vi "f_6_Eon.vi"(0 "file path (IN)":path, 1 "Project #":string, 2 "Request #":string, 3 "TEST #":string, 5 "error in (no error)":errorcluster, 6 "VGE":dbl, 8 "VCE":dbl) -> (14 "file path (OUT)":path, 15 "Eon (uj)":dbl, 16 "DONE Eon":bool, 19 "error out":errorcluster)   [LabVIEW 2020]
uses:
  GlobIndSw1.vi
  <vilib>/Waveform/WDTOps.llb/WDT Waveform Duration DBL.vi
  <vilib>/Waveform/WDTOps.llb/WDT Get Waveform Subset DBL.vi
  <vilib>/measure/mamon.llb/Trigger Detection for 1 Channel.vi
  <vilib>/Analysis/NI_AALBase.lvlib
  <vilib>/measure/NI_MAPro.lvlib
panel:
  in  "Decision ?":bool
  out "Cursor a : Channel 3":dbl
  out "Cursor a : Channel 2":dbl
  out "3% Vce":dbl
  out "10% Vge":dbl
  out "Waveform Graph":waveform(dbl)[](graph)
  out "ON Region":waveform(dbl)[](graph) caption="Eon (uj)"
  out "Eon Area X-axis":dbl[](array[numeric])
  out "Eon : XY Graph":cluster{"X":dbl, "Y":dbl}[](graph)
  out "Eon Area Y-axis":dbl[](array[numeric])
  # "Eon =  from 10% Vge to 3% Vce"
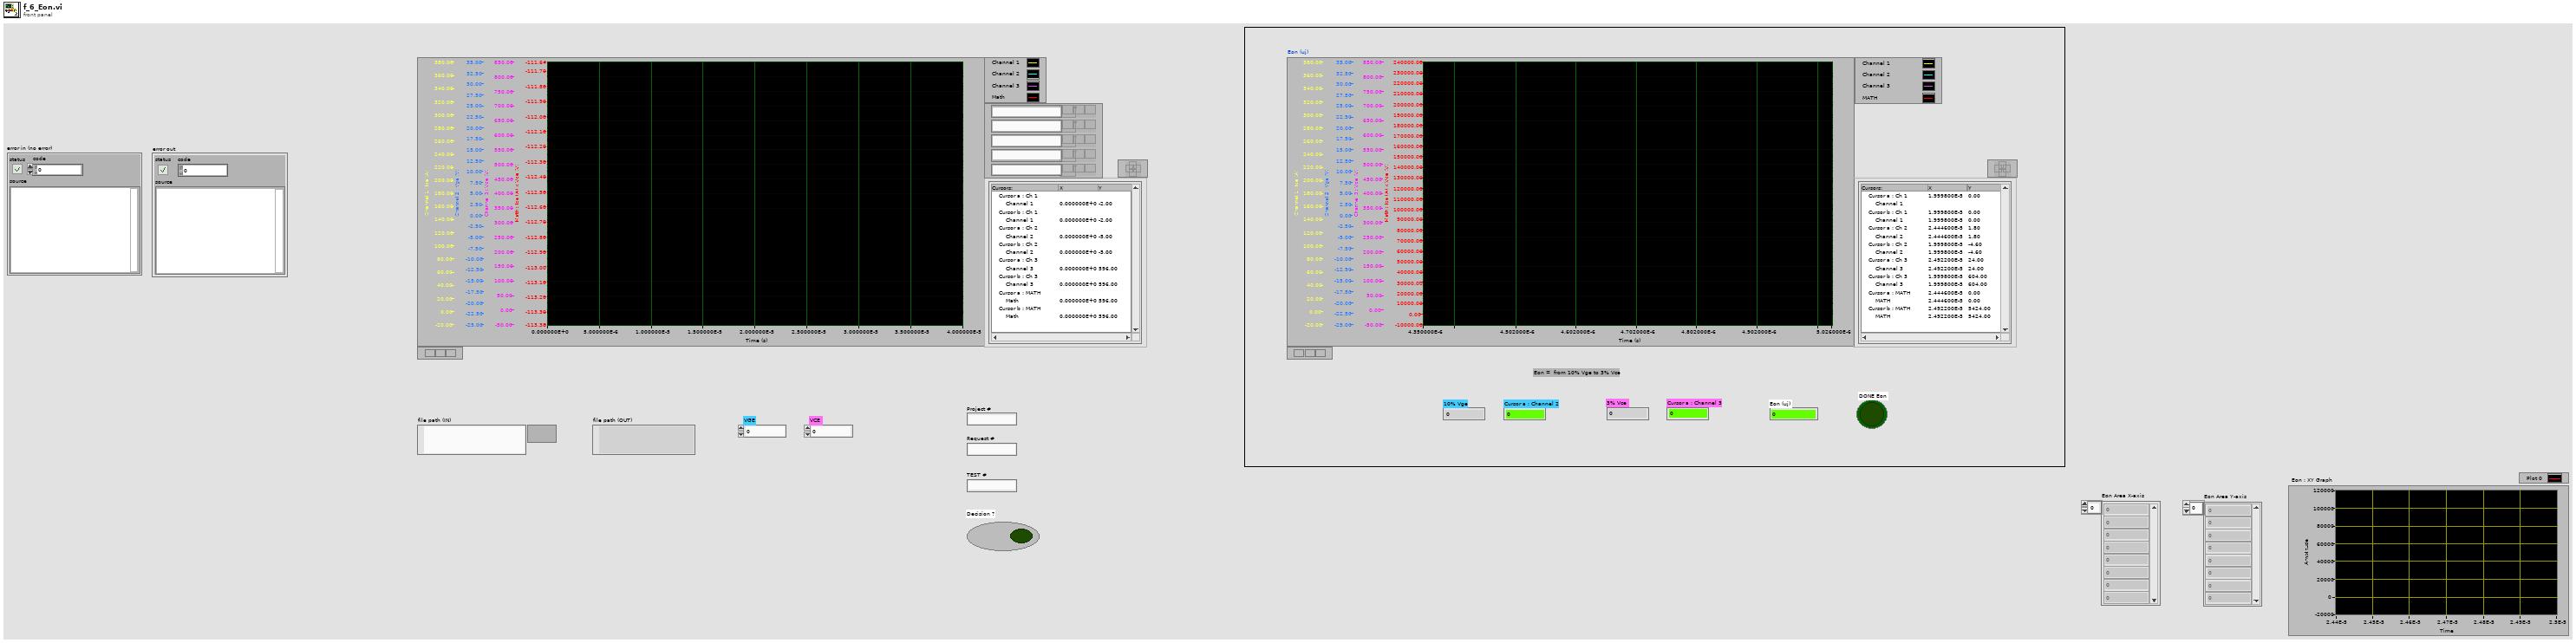
[diagram p1: front panel]
types:
  T1 = enum32{"Invalid", "Standard", "Closed", "Hidden", "Minimized", "Maximized"}
  T2 = typedef "imagedata.ctl" = cluster{"image type":i32, "image depth":i32, "image":u8[], "mask":u8[], "colors":u32[], "Rectangle":cluster{"left":i16, "top":i16, "right":i16, "bottom":i16}}
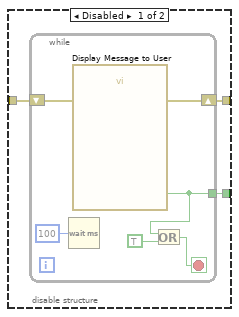
[diagram p3: hidden frame]
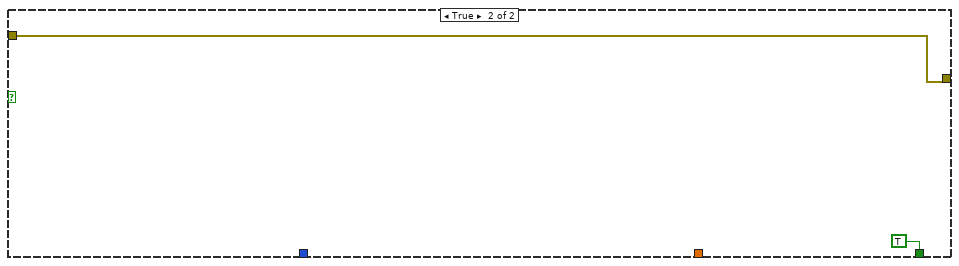
[diagram p10: hidden frame]
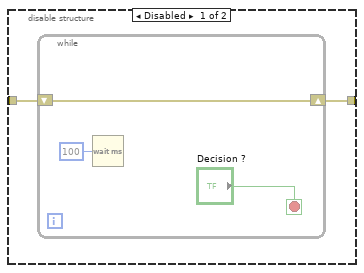
[diagram p11: hidden frame]
diagram:
  w1 = 0.0 ("Eon (uj)")
  w6 = errorcluster {"status"=FALSE, "code"=0, "source"=""} ("error out")
  w2 = FALSE ("DONE Tdon")
  w7 = waveform(dbl)[] [] ("Waveform Graph")
  n1 = local write "Eon (uj)"(w1) -> ()
  n2 = local write "Cursor a : Channel 2"(w1) -> ()
  n3 = local write "Cursor a : Channel 3"(w1) -> ()
  n4 = local write "DONE Eon"(w2) -> ()
  n5 = local write "Decision ?"(w2) -> ()
  n6 = local write "error out"(w6) -> ()
  n7 = local write "error in (no error)"(w6) -> ()
  n8 = local write "Waveform Graph"(w7) -> ()
  n9 = local write "ON Region"(w7) -> ()
  n10 = disable-structure shown="Disabled" {
    frame Disabled {
      n11 = control-ref of="This VI"() -> (w15:refnum<vi>)
      n12 = invoke class="VI" method="FP.Close"() -> (reference=w14:refnum<vi>)  [unwired: 2 in, 3 out]
      n13 = invoke class="VI" method="FP.Open"(reference=w15, "Activate"=TRUE ("Activate?"), "State"=T1."Maximized") -> (error in=w18:errorcluster, error out=w16:errorcluster)  [unwired: 1 in, 4 out]
      n14 = property class="VI"(reference=w15, error in=w16, "Front Panel.Closeable"=TRUE ("Front Panel Window:Closeable")) -> ()  [unwired: 2 out]
    }
    frame Enabled {
    }
  }
  n15 = flat-sequence {
    tunnel: ["file path (IN)"] -> w13
    tunnel: [w21] -> w12
    tunnel: [w32] -> w11
    tunnel: [w31] -> w10
    tunnel: w13 -> [w30]
    tunnel: w12 -> [w29]
    tunnel: w11 -> [w432]
    tunnel: [w431] -> w9
    tunnel: [w430] -> w8
    tunnel: w10 -> [w430]
    tunnel: w9 -> [w445]
    tunnel: w8 -> [w446]
    frame #0 {
      n16 = control-ref of="This VI"() -> (w23:refnum<vi>)
      n17 = invoke class="VI" method="FP.Open"(reference=w23, error in="error in (no error)", "Activate"=TRUE ("Activate?"), "State"=T1."Maximized") -> (error out=w24:errorcluster)  [unwired: 1 in, 4 out]
      n18 = property class="VI"(reference=w23, error in=w24, "Front Panel.Closeable"=TRUE ("Front Panel Window:Closeable")) -> (error out=w21:errorcluster)  [unwired: 1 out]
    }
    frame #1 {
      n19 = while {
        shift-right: [w39] -> w32
        shift-left: w29 -> [w37]
        tunnel: [w35] -> w31
        tunnel: w30 -> [w34]
        stop <- w40 stop-if-true
        n20 = flat-sequence {
          tunnel: w37 -> [w86]
          tunnel: [w86] -> w38
          tunnel: w34 -> [w79]
          tunnel: [w79] -> w33
          tunnel: [w90] -> w66
          tunnel: [w89] -> w65
          tunnel: [w113] -> w64
          tunnel: [w103] -> w63
          tunnel: [w97] -> w62
          tunnel: w38 -> [w186]
          tunnel: w33 -> [w181]
          tunnel: w66 -> [w265]
          tunnel: w65 -> [w259]
          tunnel: w64 -> [w258]
          tunnel: [w274] -> w61
          tunnel: w63 -> [w273]
          tunnel: [w273] -> w60
          tunnel: [w256] -> w59
          tunnel: [w264] -> w58
          tunnel: w62 -> [w270]
          tunnel: [w270] -> w57
          tunnel: w61 -> [w298]
          tunnel: [w295] -> w56
          tunnel: w60 -> [w304]
          tunnel: [w304] -> w55
          tunnel: w59 -> [w303]
          tunnel: [w303] -> w54
          tunnel: w58 -> [w302]
          tunnel: [w302] -> w53
          tunnel: w57 -> [w301]
          tunnel: [w301] -> w52
          tunnel: w56 -> [w316]
          tunnel: [w311] -> w51
          tunnel: w55 -> [w317]
          tunnel: [w317] -> w50
          tunnel: w54 -> [w307]
          tunnel: [w307] -> w49
          tunnel: w53 -> [w308]
          tunnel: [w308] -> w48
          tunnel: w52 -> [w315]
          tunnel: w51 -> [w399]
          tunnel: [w398] -> w47
          tunnel: w50 -> [w406]
          tunnel: [w406] -> w46
          tunnel: w49 -> [w395]
          tunnel: w48 -> [w394]
          tunnel: [w394] -> w45
          tunnel: [w395] -> w44
          tunnel: w47 -> [w418]
          tunnel: [w417] -> w43
          tunnel: w46 -> [w419]
          tunnel: [w419] -> w42
          tunnel: w45 -> [w412]
          tunnel: w44 -> [w411]
          tunnel: w43 -> [w422]
          tunnel: w42 -> [w420]
          tunnel: [w421] -> w41
          tunnel: [w420] -> w35
          frame #0 {
            w85 = waveform(dbl)[] [] ("Waveform Graph")
            w81 = 0.0 ("Eon (uj)")
            w80 = FALSE ("DONE Tdon")
            n21 = local write "Eon (uj)"(w81) -> ()
            n22 = local write "Cursor a : Channel 2"(w81) -> ()
            n23 = local write "Cursor a : Channel 3"(w81) -> ()
            n24 = local write "DONE Eon"(w80) -> ()
            n25 = local write "Decision ?"(w80) -> ()
            n26 = Wait (ms)(milliseconds to wait=u32 400) -> ()  [unwired: 1 out]
            n27 = local write "Eon Area X-axis"(dbl[] [] ("Eon Area X-axis")) -> ()
            n28 = local write "Eon : XY Graph"(cluster{"X":dbl, "Y":dbl}[] [] ("Eon : XY Graph")) -> ()
            n29 = local write "Eon Area Y-axis"(dbl[] [] ("Eon Area X-axis")) -> ()
            n30 = local write "Waveform Graph"(w85) -> ()
            n31 = local write "ON Region"(w85) -> ()
          }
          frame #1 {
            w163 = u16 1 items=["Samples", "Relative Time"] ("start/duration format")
            w173 = u16 1 items=["Samples", "Relative Time"] ("start/duration format")
            w174 = u16 1 items=["Samples", "Relative Time"] ("start/duration format")
            # "Channel 1"
            # "Channel 3"
            # "Channel 2"
            # "dt"
            # "Ch2"
            # "Ch1"
            n32 = call "3_ReadDatatoWaveform.vi"("error in (no error)"=w186, "file path (IN)"=w181) -> ("error out"=w95:errorcluster, "Waveform Graph"=→"Waveform Graph":waveform(dbl)[], "file path (OUT)"=w103:path, "dt"=w182:dbl, "Ch 2 Data"=w179:dbl[], "Ch 3 Data"=w183:dbl[], "Ch 1 Data"=w180:dbl[])  [unwired: 3 in]
            n33 = To Time Stamp(1:0.0 ("number")) -> (0:w184:timestamp)
            n34 = Wait (ms)(milliseconds to wait=u32 400) -> ()  [unwired: 1 out]
            n35 = call <vilib>:"Beep.vi"("use system alert? (T)"=FALSE, "duration (msec)"=u32 200, "frequency (Hz)"=u32 2000) -> ()  [unwired: 9 in]
            n36 = disable-structure shown="Enabled" {
              disable-tunnel: w184 -> [w248 _]
              disable-tunnel: w182 -> [w247 _]
              disable-tunnel: w183 -> [w246 _]
              disable-tunnel: [w245 _] -> w93
              frame Enabled {
                # "Channel 3"
                n37 = Bundle By Name("Y"=w246, "dt"=w247, "t0"=w248) -> (w245:waveform(dbl))  [unwired: 1 in]
              }
              frame Disabled {
              }
            }
            n38 = disable-structure shown="Enabled" {
              disable-tunnel: w184 -> [w244 _]
              disable-tunnel: w182 -> [w243 _]
              disable-tunnel: w179 -> [w242 _]
              disable-tunnel: [w241 _] -> w94
              frame Enabled {
                # "Channel 2"
                n39 = Bundle By Name("Y"=w242, "dt"=w243, "t0"=w244) -> (w241:waveform(dbl))  [unwired: 1 in]
              }
              frame Disabled {
              }
            }
            n40 = disable-structure shown="Enabled" {
              disable-tunnel: w184 -> [w240 _]
              disable-tunnel: w182 -> [w239 _]
              disable-tunnel: w180 -> [w238 _]
              disable-tunnel: [w237 _] -> w100
              frame Enabled {
                # "Channel 1"
                n41 = Bundle By Name("Y"=w238, "dt"=w239, "t0"=w240) -> (w237:waveform(dbl))  [unwired: 1 in]
              }
              frame Disabled {
              }
            }
            n42 = global read "GlobIndSw1.vi" "Median Filter Rank"() -> (w88:i32)
            n43 = disable-structure shown="Enabled" {
              disable-tunnel: w93 -> [w198 _]
              disable-tunnel: [w190 _] -> w91
              disable-tunnel: [w189 _] -> w89
              disable-tunnel: w95 -> [w188 _]
              disable-tunnel: w88 -> [w187 _]
              frame Enabled {
                w192 = u16 1 items=["Samples", "Relative Time"] ("start/duration format")
                # "Channel 3 - Filtered"
                # "Median"
                n44 = Unbundle By Name(w198) -> ("Y"=w201:dbl[], "dt"=w199:dbl)
                n45 = call <vilib>:"Median Filter.vi"("right rank"=w187, "left rank"=w187, "X"=w201) -> ("Filtered X"=w200:dbl[])  [unwired: 7 in, 1 out]
                n46 = Bundle By Name("Y"=w200, "dt"=w199) -> (w191:waveform(dbl))  [unwired: 1 in]
                n47 = call-poly <vilib>:"Waveform Duration.vi"("error in (no error)"=w188, "waveform in"=w191) -> ("error out"=w195:errorcluster, "duration"=w197:dbl, "waveform out"=w196:waveform(dbl))  [unwired: 7 in]
                n48 = Divide(x=w197, y=2.0) -> (x/y=w194:dbl)
                n49 = call-poly <vilib>:"Get Waveform Subset.vi"("start/duration format"=w192, "error in (no error)"=w195, "duration"=w194, "start samples/time"=w194, "waveform in"=w196) -> ("error out"=w190:errorcluster, "waveform out"=w189:waveform(dbl))  [unwired: 1 in, 2 out]
              }
              frame Disabled {
              }
            }
            n50 = disable-structure shown="Enabled" {
              disable-tunnel: w94 -> [w213 _]
              disable-tunnel: [w205 _] -> w92
              disable-tunnel: [w204 _] -> w90
              disable-tunnel: w95 -> [w203 _]
              disable-tunnel: w88 -> [w202 _]
              frame Enabled {
                w207 = u16 1 items=["Samples", "Relative Time"] ("start/duration format")
                # "Channel 2 - Filtered"
                # "Median"
                n51 = Unbundle By Name(w213) -> ("Y"=w216:dbl[], "dt"=w214:dbl)
                n52 = call <vilib>:"Median Filter.vi"("right rank"=w202, "left rank"=w202, "X"=w216) -> ("Filtered X"=w215:dbl[])  [unwired: 7 in, 1 out]
                n53 = Bundle By Name("Y"=w215, "dt"=w214) -> (w206:waveform(dbl))  [unwired: 1 in]
                n54 = call-poly <vilib>:"Waveform Duration.vi"("error in (no error)"=w203, "waveform in"=w206) -> ("error out"=w210:errorcluster, "duration"=w212:dbl, "waveform out"=w211:waveform(dbl))  [unwired: 7 in]
                n55 = Divide(x=w212, y=2.0) -> (x/y=w209:dbl)
                n56 = call-poly <vilib>:"Get Waveform Subset.vi"("start/duration format"=w207, "error in (no error)"=w210, "duration"=w209, "start samples/time"=w209, "waveform in"=w211) -> ("error out"=w205:errorcluster, "waveform out"=w204:waveform(dbl))  [unwired: 1 in, 2 out]
              }
              frame Disabled {
              }
            }
            n57 = disable-structure shown="Enabled" {
              disable-tunnel: w100 -> [w233 _]
              disable-tunnel: w93 -> [w232 _]
              disable-tunnel: [w220 _] -> w98
              disable-tunnel: [w219 _] -> w97
              disable-tunnel: w95 -> [w217 _]
              frame Enabled {
                w226 = u16 1 items=["Samples", "Relative Time"] ("start/duration format")
                # "Channel 3"
                # "Channel 1"
                # "Channel MATH"
                # "MATH = Ch1 x Ch3"
                n58 = Unbundle By Name(w232) -> ("Y"=w229:dbl[])
                n59 = Unbundle By Name(w233) -> ("Y"=w230:dbl[], "dt"=w218:dbl, "t0"=w231:timestamp)
                n60 = for {
                  tunnel: w230 -> [w236] mode=indexing
                  tunnel: w229 -> [w235] mode=indexing
                  tunnel: [w234] -> w228 mode=indexing
                  n61 = Multiply(x=w236, y=w235) -> (x*y=w234:dbl)
                }
                n62 = Bundle By Name("Y"=w228, "dt"=w218, "t0"=w231) -> (w221:waveform(dbl))  [unwired: 1 in]
                n63 = call-poly <vilib>:"Waveform Duration.vi"("error in (no error)"=w217, "waveform in"=w221) -> ("error out"=w222:errorcluster, "duration"=w224:dbl, "waveform out"=w227:waveform(dbl))  [unwired: 7 in]
                n64 = Divide(x=w224, y=2.0) -> (x/y=w225:dbl)
                n65 = call-poly <vilib>:"Get Waveform Subset.vi"("start/duration format"=w226, "error in (no error)"=w222, "duration"=w225, "start samples/time"=w225, "waveform in"=w227) -> ("error out"=w220:errorcluster, "waveform out"=w219:waveform(dbl))  [unwired: 1 in, 2 out]
              }
              frame Disabled {
              }
            }
            n66 = call-poly <vilib>:"Waveform Duration.vi"("error in (no error)"=w95, "waveform in"=w100) -> ("error out"=w178:errorcluster, "duration"=w175:dbl, "waveform out"=w177:waveform(dbl))  [unwired: 7 in]
            n67 = call-poly <vilib>:"Waveform Duration.vi"("error in (no error)"=w95, "waveform in"=w94) -> ("error out"=w168:errorcluster, "duration"=w171:dbl, "waveform out"=w169:waveform(dbl))  [unwired: 7 in]
            n68 = call-poly <vilib>:"Waveform Duration.vi"("error in (no error)"=w95, "waveform in"=w93) -> ("error out"=w167:errorcluster, "duration"=w165:dbl, "waveform out"=w101:waveform(dbl))  [unwired: 7 in]
            n69 = Divide(x=w175, y=2.0) -> (x/y=w161:dbl)
            n70 = Divide(x=w171, y=2.0) -> (x/y=w172:dbl)
            n71 = Divide(x=w165, y=2.0) -> (x/y=w164:dbl)
            n72 = call-poly <vilib>:"Get Waveform Subset.vi"("start/duration format"=w174, "error in (no error)"=w178, "duration"=w161, "start samples/time"=w161, "waveform in"=w177) -> ("error out"=w160:errorcluster, "waveform out"=w114:waveform(dbl))  [unwired: 1 in, 2 out]
            n73 = call-poly <vilib>:"Get Waveform Subset.vi"("start/duration format"=w173, "error in (no error)"=w168, "duration"=w172, "start samples/time"=w172, "waveform in"=w169) -> ("error out"=w159:errorcluster, "waveform out"=w115:waveform(dbl))  [unwired: 1 in, 2 out]
            n74 = call-poly <vilib>:"Get Waveform Subset.vi"("start/duration format"=w163, "error in (no error)"=w167, "duration"=w164, "start samples/time"=w164, "waveform in"=w101) -> ("error out"=w96:errorcluster, "waveform out"=w102:waveform(dbl))  [unwired: 1 in, 2 out]
            n75 = Build Array(w114, w115, w102, w97) -> (→"ON Region":waveform(dbl)[])
            n76 = Merge Errors(w160, w159, w96, w98, w92, w91) -> (w111:errorcluster)
            n77 = property on="ON Region" class="WFGraph (strict)"(error in=w111) -> (error out=w110:errorcluster, "Width"=w109:u32)  [unwired: 1 in, 1 out]
            n78 = property on="ON Region" class="WFGraph (strict)"(error in=w110, "Caption.Justify"=enum16{"Left", "Center", "Right"}."Left" ("Caption.Justification"), "Caption.Width"=w109, "Caption.FontBold"=TRUE ("Caption.Font:Bold"), "Caption.FontColor"=u32 16860 ("Caption.Font:Color"), "Caption.FontSize"=u32 24 ("Caption.Font:Size"), "Caption.Text"="Eon (uj)") -> (error out=w105:errorcluster)  [unwired: 1 in, 1 out]
            n79 = property on="ON Region" class="WFGraph (strict)"(error in=w105, "XScale.Offset"=w161) -> (error out=w139:errorcluster)  [unwired: 1 in, 1 out]
            n80 = property on="ON Region" class="WFGraph (strict)"(error in=w139, "Active Cursor"=u32 0, "Cursor.Cursor X"=0.0 ("Cursor.Cursor Position:Cursor X"), "Cursor.Cursor Y"=0.0 ("Cursor.Cursor Position:Cursor Y"), "Cursor.Visible"=FALSE) -> (error out=w138:errorcluster)  [unwired: 1 in, 1 out]
            n81 = property on="ON Region" class="WFGraph (strict)"(error in=w138, "Active Cursor"=u32 1, "Cursor.Cursor X"=0.0 ("Cursor.Cursor Position:Cursor X"), "Cursor.Cursor Y"=0.0 ("Cursor.Cursor Position:Cursor Y"), "Cursor.Visible"=FALSE) -> (error out=w137:errorcluster)  [unwired: 1 in, 1 out]
            n82 = property on="ON Region" class="WFGraph (strict)"(error in=w137, "Active Cursor"=u32 2, "Cursor.Cursor X"=0.0 ("Cursor.Cursor Position:Cursor X"), "Cursor.Cursor Y"=0.0 ("Cursor.Cursor Position:Cursor Y"), "Cursor.Visible"=FALSE) -> (error out=w136:errorcluster)  [unwired: 1 in, 1 out]
            n83 = property on="ON Region" class="WFGraph (strict)"(error in=w136, "Active Cursor"=u32 3, "Cursor.Cursor X"=0.0 ("Cursor.Cursor Position:Cursor X"), "Cursor.Cursor Y"=0.0 ("Cursor.Cursor Position:Cursor Y"), "Cursor.Visible"=FALSE) -> (error out=w119:errorcluster)  [unwired: 1 in, 1 out]
            n84 = property on="ON Region" class="WFGraph (strict)"(error in=w119, "Active Cursor"=u32 4, "Cursor.Cursor X"=0.0 ("Cursor.Cursor Position:Cursor X"), "Cursor.Cursor Y"=0.0 ("Cursor.Cursor Position:Cursor Y"), "Cursor.Visible"=FALSE) -> (error out=w118:errorcluster)  [unwired: 1 in, 1 out]
            n85 = property on="ON Region" class="WFGraph (strict)"(error in=w118, "Active Cursor"=u32 5, "Cursor.Cursor X"=0.0 ("Cursor.Cursor Position:Cursor X"), "Cursor.Cursor Y"=0.0 ("Cursor.Cursor Position:Cursor Y"), "Cursor.Visible"=FALSE) -> (error out=w117:errorcluster)  [unwired: 1 in, 1 out]
            n86 = property on="ON Region" class="WFGraph (strict)"(error in=w117, "Active Cursor"=u32 6, "Cursor.Cursor X"=0.0 ("Cursor.Cursor Position:Cursor X"), "Cursor.Cursor Y"=0.0 ("Cursor.Cursor Position:Cursor Y"), "Cursor.Visible"=FALSE) -> (error out=w116:errorcluster)  [unwired: 1 in, 1 out]
            n87 = property on="ON Region" class="WFGraph (strict)"(error in=w116, "Active Cursor"=u32 7, "Cursor.Cursor X"=0.0 ("Cursor.Cursor Position:Cursor X"), "Cursor.Cursor Y"=0.0 ("Cursor.Cursor Position:Cursor Y"), "Cursor.Visible"=FALSE) -> (error out=w113:errorcluster)  [unwired: 1 in, 1 out]
          }
          frame #2 {
            w262 = u16 0 items=["Falling Edge", "Rising Edge"] ("trigger slope")
            w263 = u16 1 items=["Index", "Time"] ("location mode")
            w268 = u16 1 items=["Falling Edge", "Rising Edge"] ("trigger slope")
            w269 = u16 1 items=["Index", "Time"] ("location mode")
            # "Cursor a : Channel 2"
            # "Cursor a : Channel 3"
            # "End Time 2nd Cursor"
            # "End Time 1st Cursor"
            # "2nd PARAMETER"
            # "Channel 3"
            # "1st PARAMETER"
            # "Channel 2"
            n88 = Wait (ms)(milliseconds to wait=u32 500) -> ()  [unwired: 1 out]
            n89 = call <vilib>:"Beep.vi"("use system alert? (T)"=FALSE, "duration (msec)"=u32 200, "frequency (Hz)"=u32 2000) -> ()  [unwired: 9 in]
            n90 = Divide(x=3.0, y=100.0) -> (x/y=w291:dbl)
            n91 = Divide(x=10.0, y=100.0) -> (x/y=w287:dbl)
            n92 = Multiply(x=w291, y="VCE") -> (x*y=w260:dbl)
            "3% Vce" <- w260
            n93 = Multiply(x=w287, y="VGE") -> (x*y=w266:dbl)
            "10% Vge" <- w266
            n94 = Add(x=w260, y=0.2) -> (x+y=w251:dbl)
            n95 = Add(x=w266, y=0.2) -> (x+y=w255:dbl)
            n96 = Divide(x=w251, y=10.0) -> (x/y=w250:dbl)
            n97 = Divide(x=w255, y=10.0) -> (x/y=w253:dbl)
            n98 = call-poly <vilib>:"Basic Level Trigger Detection.vi"("signal in"=w259, "level"=w251, "hysteresis"=w250, "location mode"=w263, "error in (no error)"=w258, "trigger slope"=w262) -> ("trigger location"=w256:dbl, "error out"=w257:errorcluster)  [unwired: 7 in, 1 out]
            n99 = call-poly <vilib>:"Basic Level Trigger Detection.vi"("signal in"=w265, "level"=w255, "hysteresis"=w253, "location mode"=w269, "trigger slope"=w268) -> ("trigger location"=w264:dbl)  [unwired: 8 in, 2 out]
            n100 = property on="ON Region" class="WFGraph (strict)"(error in=w258, "Active Cursor"=u32 2, "Cursor.Cursor X"=w264, "Cursor.Visible"=TRUE, "Cursor.Cursor Name Visible"=TRUE) -> (error out=w275:errorcluster)  [unwired: 1 in, 1 out]
            n101 = property on="ON Region" class="WFGraph (strict)"(error in=w257, "Active Cursor"=u32 4, "Cursor.Cursor X"=w256, "Cursor.Visible"=TRUE, "Cursor.Cursor Name Visible"=TRUE) -> (error out=w276:errorcluster)  [unwired: 1 in, 1 out]
            n102 = Merge Errors(w276, w275) -> (w274:errorcluster)
          }
          frame #3 {
            # "Cursor a : Channel 3"
            # "Cursor a : Channel 2"
            n103 = property on="ON Region" class="WFGraph (strict)"(error in=w298, "Active Cursor"=u32 4) -> (error out=w297:errorcluster, "Cursor.Cursor Y"=→"Cursor a : Channel 3":dbl)  [unwired: 1 in, 1 out]
            n104 = property on="ON Region" class="WFGraph (strict)"(error in=w298, "Active Cursor"=u32 2) -> (error out=w296:errorcluster, "Cursor.Cursor Y"=→"Cursor a : Channel 2":dbl)  [unwired: 1 in, 1 out]
            n105 = Wait (ms)(milliseconds to wait=u32 300) -> ()  [unwired: 1 out]
            n106 = Merge Errors(w297, w296) -> (w295:errorcluster)
          }
          frame #4 {
            # "https://forums.ni.com/t5/LabVIEW/area-under-curve-of-an-XY-graph-with-constant-non-equi-distant-x/m-p/254797?profile.language=en&query.id=125746#M137523"
            n107 = flat-sequence {
              tunnel: w316 -> [w323]
              tunnel: w307 -> [w322]
              tunnel: w308 -> [w321]
              tunnel: [w318] -> w314
              tunnel: w314 -> [w332]
              tunnel: w309 -> [w331]
              tunnel: [w330] -> w313
              tunnel: w313 -> [w376]
              tunnel: [w376] -> w312
              tunnel: [w374] -> w310
              tunnel: [w373] -> w306
              tunnel: [w392] -> w311
              tunnel: w312 -> [w392]
              tunnel: w310 -> [w382]
              tunnel: w306 -> [w383]
              frame #0 {
                # "Cursor b : MATH"
                # "Cursor a : MATH"
                n108 = property on="ON Region" class="WFGraph (strict)"(error in=w323, "Active Cursor"=u32 6, "Cursor.Cursor X"=w321, "Cursor.Visible"=TRUE, "Cursor.Cursor Name Visible"=TRUE) -> (error out=w319:errorcluster)  [unwired: 1 in, 1 out]
                n109 = property on="ON Region" class="WFGraph (strict)"(error in=w323, "Active Cursor"=u32 7, "Cursor.Cursor X"=w322, "Cursor.Visible"=TRUE, "Cursor.Cursor Name Visible"=TRUE) -> (error out=w320:errorcluster)  [unwired: 1 in, 1 out]
                n110 = Merge Errors(w320, w319) -> (w318:errorcluster)
              }
              frame #1 {
                n111 = while {
                  tunnel: w332 -> [w340]
                  tunnel: w331 -> [w337]
                  tunnel: [w334] -> w330
                  i -> [w339]
                  stop <- w341 stop-if-true
                  # "Cursor b : MATH"
                  # "Cursor a : MATH"
                  n112 = property on="ON Region" class="WFGraph (strict)"(error in=w340, "Active Cursor"=u32 7) -> (error out=w336:errorcluster, "Cursor.Cursor X"=w343:dbl)  [unwired: 1 in, 1 out]
                  n113 = property on="ON Region" class="WFGraph (strict)"(error in=w340, "Active Cursor"=u32 6) -> (error out=w338:errorcluster, "Cursor.Cursor X"=w345:dbl)  [unwired: 1 in, 1 out]
                  n114 = Merge Errors(w338, w336) -> (w335:errorcluster)
                  n115 = Equal?(x=w345, y=w343) -> (x = y?=w342:bool)
                  n116 = case shown="False" w342 {
                    tunnel: [FALSE ("Cursor.Visible") TRUE ("Cursor.Visible")] -> w341
                    tunnel: w339 -> [w351 _]
                    tunnel: w337 -> [w350 _]
                    tunnel: w335 -> [w349 w371]
                    tunnel: [w347 w371] -> w334
                    frame False {
                      n117 = flat-sequence {
                        tunnel: w351 -> [w357]
                        tunnel: w349 -> [w354]
                        tunnel: [w353] -> w348
                        tunnel: w350 -> [w367]
                        tunnel: w348 -> [w365]
                        tunnel: [w363] -> w347
                        frame #0 {
                          # "Cursor a : MATH"
                          n118 = property on="ON Region" class="WFGraph (strict)"(error in=w354, "Active Cursor"=u32 6) -> (error out=w353:errorcluster, "Cursor.Cursor X"=w356:dbl, "Cursor.Cursor Y"=w355:dbl)  [unwired: 1 in, 1 out]
                          n119 = local read "Eon Area Y-axis"() -> (w360:dbl[])
                          n120 = local read "Eon Area X-axis"() -> (w361:dbl[])
                          n121 = Insert Into Array(array=w360, index=w357, new element=w355) -> (w358:dbl[])
                          n122 = Insert Into Array(array=w361, index=w357, new element=w356) -> (w359:dbl[])
                          n123 = local write "Eon Area X-axis"(w359) -> ()
                          n124 = local write "Eon Area Y-axis"(w358) -> ()
                        }
                        frame #1 {
                          # "Cursor a : MATH"
                          # "Cursor a : MATH"
                          n125 = property on="ON Region" class="WFGraph (strict)"(error in=w365, "Active Cursor"=u32 6) -> (error out=w364:errorcluster, "Cursor.Cursor X"=w368:dbl)  [unwired: 1 in, 1 out]
                          n126 = Add(x=w368, y=w367) -> (x+y=w366:dbl)
                          n127 = property on="ON Region" class="WFGraph (strict)"(error in=w364, "Active Cursor"=u32 6, "Cursor.Cursor X"=w366) -> (error out=w363:errorcluster)  [unwired: 1 in, 1 out]
                        }
                      }
                    }
                    frame True {
                    }
                  }
                  n128 = Wait (ms)(milliseconds to wait=u32 1) -> ()  [unwired: 1 out]
                }
              }
              frame #2 {
                n129 = local read "Eon Area Y-axis"() -> (w373:dbl[])
                n130 = local read "Eon Area X-axis"() -> (w374:dbl[])
                n131 = Build Cluster Array(w374, w373) -> (w377:cluster{dbl, dbl}[])
                n132 = local write "Eon : XY Graph"(w377) -> ()
                n133 = Wait (ms)(milliseconds to wait=u32 50) -> ()  [unwired: 1 out]
              }
              frame #3 {
                n134 = Wait (ms)(milliseconds to wait=u32 50) -> ()  [unwired: 1 out]
                n135 = Delete From Array(array=w382, index=0) -> (array with subset deleted=w391:dbl[])  [unwired: 1 in, 1 out]
                n136 = Delete From Array(array=w383, index=0) -> (array with subset deleted=w385:dbl[])  [unwired: 1 in, 1 out]
                n137 = Subtract(x=w391, y=w382) -> (x-y=w390:dbl[])
                n138 = Add(x=w385, y=w383) -> (x+y=w389:dbl[])
                n139 = Compound Arithmetic op=MULTIPLY(w390, w389, invert 2.0 ("Numeric")) -> (w387:dbl[])
                n140 = Add Array Elements(numeric array=w387) -> (sum=w380:dbl)
                n141 = Multiply(x=w380, y=1000000.0) -> (x*y=→"Eon (uj)":dbl)
              }
            }
            n142 = Unbundle By Name(w315) -> ("dt"=w309:dbl)
            n143 = Wait (ms)(milliseconds to wait=u32 400) -> ()  [unwired: 1 out]
          }
          frame #5 {
            # "Cursor a : MATH"
            # "Cursor b : MATH"
            n144 = property on="ON Region" class="WFGraph (strict)"(error in=w399, "Active Cursor"=u32 7, "Cursor.Cursor X"=w395, "Cursor.Visible"=TRUE, "Cursor.Cursor Name Visible"=TRUE) -> (error out=w396:errorcluster)  [unwired: 1 in, 1 out]
            n145 = property on="ON Region" class="WFGraph (strict)"(error in=w399, "Active Cursor"=u32 6, "Cursor.Cursor X"=w394, "Cursor.Visible"=TRUE, "Cursor.Cursor Name Visible"=TRUE) -> (error out=w397:errorcluster)  [unwired: 1 in, 1 out]
            n146 = Wait (ms)(milliseconds to wait=u32 300) -> ()  [unwired: 1 out]
            n147 = Merge Errors(w396, w397) -> (w398:errorcluster)
          }
          frame #6 {
            # "2nd Cursor"
            # "1st Cursor"
            n148 = Subtract(x=w412, y=1e-07) -> (x-y=w414:dbl)
            n149 = Add(x=w411, y=1e-07) -> (x+y=w413:dbl)
            n150 = property on="ON Region" class="WFGraph (strict)"(error in=w418, "XScale.Minimum"=w414, "XScale.Maximum"=w413) -> (error out=w417:errorcluster)  [unwired: 1 in, 1 out]
            n151 = Wait (ms)(milliseconds to wait=u32 300) -> ()  [unwired: 1 out]
            n152 = call <vilib>:"Beep.vi"("use system alert? (T)"=FALSE, "duration (msec)"=u32 200, "frequency (Hz)"=u32 2000) -> ()  [unwired: 9 in]
          }
          frame #7 {
            n153 = disable-structure shown="Enabled" {
              disable-tunnel: w422 -> [w424 w428]
              disable-tunnel: [w423 w428] -> w421
              frame Disabled {
                n154 = while {
                  shift-right: [w425] -> w423
                  shift-left: w424 -> [w425]
                  stop <- "Decision ?" stop-if-true
                  n155 = Wait (ms)(milliseconds to wait=u32 100) -> ()  [unwired: 1 out]
                }
              }
              frame Enabled {
              }
            }
          }
        }
        n156 = disable-structure shown="Enabled" {
          disable-tunnel: w41 -> [w69 w76]
          disable-tunnel: [w68 TRUE ("NO")] -> w40
          disable-tunnel: [w67 w76] -> w39
          frame Disabled {
            n157 = while {
              tunnel: [w71] -> w68
              shift-right: [w74] -> w67
              shift-left: w69 -> [w75]
              stop <- w73 stop-if-true
              n158 = Wait (ms)(milliseconds to wait=u32 100) -> ()  [unwired: 1 out]
              n159 = call "Display Message to User"("error in (no error)"=w75) -> ("error out"=w74:errorcluster, "NO"=w71:bool)  [unwired: 9 in]
              n160 = Or(x=w71, y=TRUE) -> (x .or. y?=w73:bool)
            }
          }
          frame Enabled {
          }
        }
        n161 = Wait (ms)(milliseconds to wait=u32 100) -> ()  [unwired: 1 out]
      }
    }
    frame #2 {
      w435 = "_"
      n162 = Wait (ms)(milliseconds to wait=u32 300) -> ()  [unwired: 1 out]
      n163 = invoke on="ON Region" class="WFGraph (strict)" method="Get Image"(error in=w432) -> (error out=w438:errorcluster, "image data"=w441:T2)  [unwired: 5 in, 4 out]
      n164 = Concatenate Strings("C:\\Inductive_Switching_Project\\IndSw_Image\\" ("string"), "Project #", w435, "Request #", w435, "TEST #", w435, "Eon" ("string"), ".png" ("string")) -> (w442:string)
      n165 = String To Path(string=w442) -> (path=w440:path)
      n166 = call <vilib>:"Write PNG File.vi"("error in (no error)"=w438, "image data"=w441, "path to PNG file"=w440) -> ("error out"=w431:errorcluster)  [unwired: 7 in, 1 out]
      "DONE Eon" <- TRUE ("DONE Tdon")
    }
    frame #3 {
      n167 = disable-structure shown="Enabled" {
        disable-tunnel: w445 -> [w447 _]
        frame Enabled {
          n168 = control-ref of="This VI"() -> (w448:refnum<vi>)
          n169 = invoke class="VI" method="FP.Close"(reference=w448, error in=w447) -> ()  [unwired: 1 in, 3 out]
        }
        frame Disabled {
        }
      }
      "file path (OUT)" <- w446
      "error out" <- w445
    }
  }
  "Eon Area Y-axis" <- dbl[] [] ("Eon Area Y-axis")
  "Eon : XY Graph" <- cluster{"X":dbl, "Y":dbl}[] [] ("Eon : XY Graph")
  "Eon Area X-axis" <- dbl[] [] ("Eon Area X-axis")
